vi "Launch Event Handle.vi"(8 "error in (no error)":errorcluster, 11 "QTab Class in":refnum<class "QTab Class.lvclass">) -> (0 "error out":errorcluster, 3 "QTab Class out":refnum<class "QTab Class.lvclass">)   [LabVIEW 2020, in "QTab.lvlib" / "QTab Class.lvclass"]
uses:
  QTab Class.lvclass
  QTab Class.lvclass/QTab Class.ctl
  Event Handle Dispatcher.vi
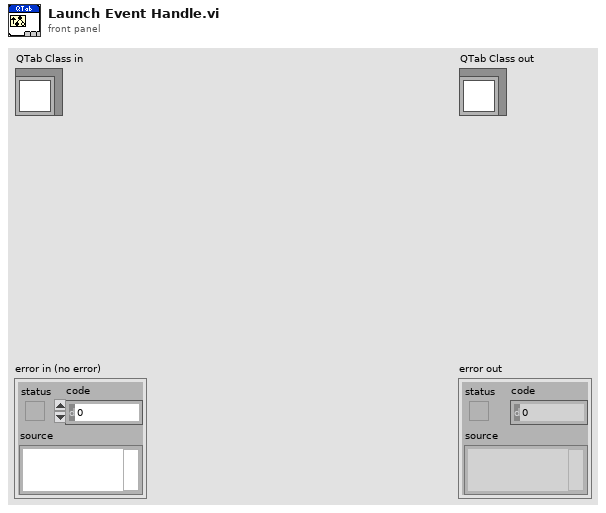
[diagram p1: front panel]
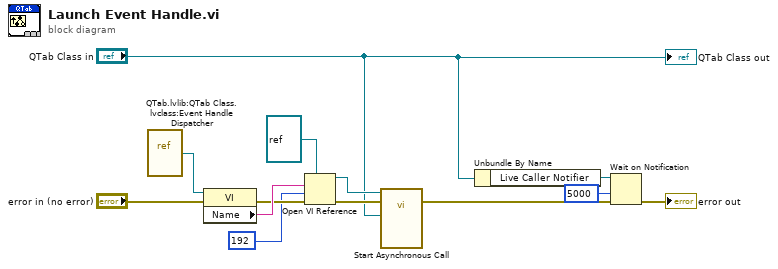
[diagram p0: block diagram]
diagram:
  n1 = vi-ref "QTab.lvlib:QTab Class.lvclass:Event Handle Dispatcher.vi"() -> (w9:refnum<vi>)
  n2 = property class="VI"(reference=w9, error in="error in (no error)") -> (error out=w12:errorcluster, "Name"=w13:string)  [unwired: 1 out]
  n3 = Open VI Reference(type specifier VI Refnum (for type only)=refnum<vi> refnum, vi path=w13, options=192, error in (no error)=w12) -> (vi reference=w7:refnum<vi>, error out=w8:errorcluster)  [unwired: 2 in]
  n4 = call-by-ref "Start Asynchronous Call"(reference=w7, error in=w8, "QTab Class in"="QTab Class in") -> (error out=w6:errorcluster)  [unwired: 10 in, 2 out]
  n5 = Unbundle By Name("QTab Class in") -> ("Live Caller Notifier"=w5:refnum<notifier>)
  n6 = Wait on Notification(notifier=w5, timeout in ms (-1)=5000, error in (no error)=w6) -> (error out=→"error out":errorcluster)  [unwired: 1 in, 3 out]
  "QTab Class out" <- "QTab Class in"
